vi "Add Name-Peroid.vi"(9 "TimePeroid(ms)":i32, 10 "Name":string, 11 "UserEventTimer in":refnum<class "TimerEngine.lvclass">) -> (3 "UserEventTimer out":refnum<class "TimerEngine.lvclass">)   [LabVIEW 2017, in "TimerEngine.lvlib" / "TimerEngine.lvclass"]
uses:
  TimerEngine.lvclass
  TimerEngine.lvclass/TimerEngine.ctl
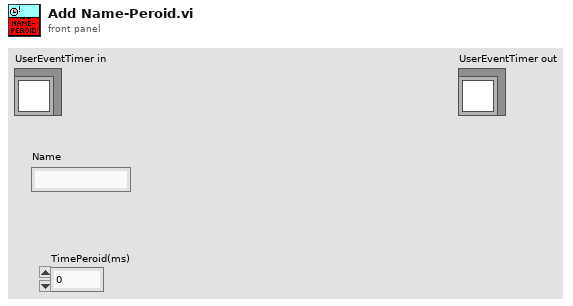
[diagram p1: front panel]
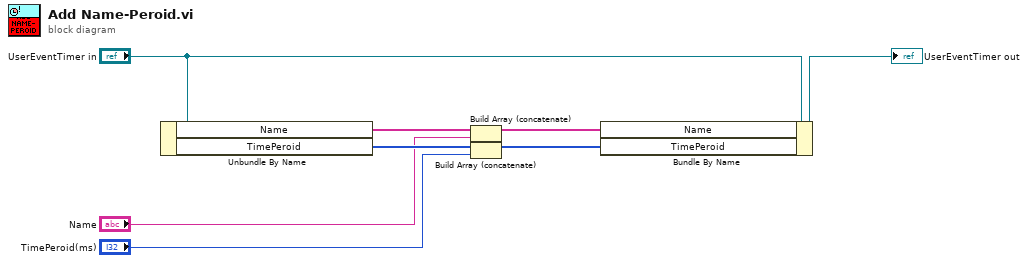
[diagram p0: block diagram]
diagram:
  n1 = Unbundle By Name("UserEventTimer in") -> ("Name"=w6:string[], "TimePeroid"=w5:i32[])
  n2 = Build Array (concatenate)(w6, "Name") -> (w4:string[])
  n3 = Build Array (concatenate)(w5, "TimePeroid(ms)") -> (w3:i32[])
  n4 = Bundle By Name(cluster="UserEventTimer in", "Name"=w4, "TimePeroid"=w3) -> (→"UserEventTimer out":refnum<class "TimerEngine.lvclass">)
